vi "ValueHasUnit.vi"() -> (0 "error out":errorcluster)   [LabVIEW 2019, in "ResultTreeTest.lvlib" / "SetDuration.lvlib"]
uses:
  55cb1a48-e70d-44f1-aae2-ae3f92a36f08.vi
  Constraint/IsEqual/Create.vi
  Constraint/IsEqual/IsEqual.lvclass
  SetDuration.lvlib
  ResultTree/ResultTree.lvclass
panel:
  in  "Tree":string(tree)
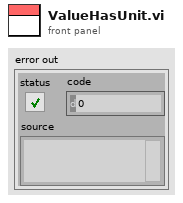
[diagram p1: front panel]
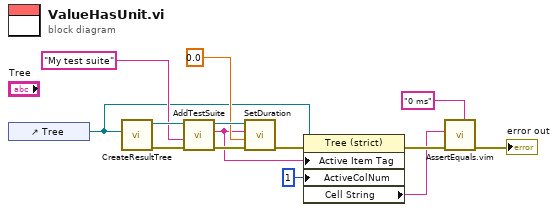
[diagram p0: block diagram]
diagram:
  n1 = control-ref of="Tree"() -> (w7:refnum<vi>)
  n2 = call "CreateResultTree.vi"("Tree Refnum"=w7) -> ("error out"=w13:errorcluster, "ResultTree out"=w12:refnum<class "ResultTree.lvclass">)  [unwired: 9 in]
  n3 = call "AddTestSuite.vi"("error in (no error)"=w13, "Name"="My test suite", "ResultTree in"=w12) -> ("error out"=w10:errorcluster, "Tag Name"=w4:string, "ResultTree out"=w9:refnum<class "ResultTree.lvclass">)  [unwired: 6 in]
  n4 = call "SetDuration.vi"("error in (no error)"=w10, "Duration [s]"=0.0, "Tag Name"=w4, "ResultTree in"=w9) -> ("error out"=w6:errorcluster)  [unwired: 6 in, 1 out]
  n5 = property class="Tree (strict)"(reference=w7, error in=w6, "Active Item Tag"=w4, "ActiveColNum"=1 ("Active Cell:Active Column Number")) -> (error out=w5:errorcluster, "Cell String"=w2:string)  [unwired: 1 out]
  n6 = call "AssertEquals.vim"("Expected"="0 ms", "error in (no error)"=w5, "Actual"=w2) -> ("error out"=→"error out":errorcluster)  [unwired: 8 in]
